vi "LV to ITX  Retrieve.vi"(0 "File or Folder Path":path=path "C:/", 5 "offset":i32, 7 "length":i32=1, 9 "index":T1={"A"=1, "B"=0, "C"=2, "D"=0, "E"=3, "N1"=0, "N2"=0, "N3"=0, "N4"=0}, 11 "stop":bool, 12 "file contains 2D data?":bool) -> (4 "A vs B":cluster{dbl[], dbl[]}[](graph)=[{[0.0624995231628418, 0.1406235694885254, 0.21874761581420898, 0.2968711853027344, 0.37499523162841797, 0.45311927795410156, 0.5468683242797852, 0.6249923706054688, 0.7031164169311523, 0.7812399864196777, 0.8593640327453613, 0.9374880790710449, 1.015612125396729, 1.109361171722412, 1.187485218048096, 1.265608787536621, 1.343732833862305, 1.437481880187988, 1.515605926513672, 1.578104972839355, 1.656229019165039, 1.749977588653564, 1.828101634979248, 1.906225681304932, 1.984349727630615, 2.062473773956299, 2.156222820281982, 2.234346389770508, 2.312470436096191, 2.390594482421875, 2.468718528747559, 2.546842575073242, 2.624966621398926, 2.703090667724609, 2.796839237213135, 2.874963283538818, 2.953087329864502, 3.031211376190186, 3.109335422515869, 3.187459468841553, 3.265583515167236, 3.359332084655762, 3.437456130981445, 3.515580177307129, 3.593704223632812, 3.671828269958496, 3.74995231628418, 3.843700885772705, 3.921824932098389, 3.999948978424072, 4.078073024749756, 4.156197071075439, 4.234321117401123, 4.312445163726807, 4.39056921005249, 4.484317779541016, 4.562441825866699, 4.640565872192383, 4.718689918518066, 4.79681396484375, 4.874938011169434, 4.968686580657959, 5.046810626983643, 5.124934673309326, 5.218683242797852, 5.296807289123535, 5.374931335449219, 5.453055381774902, 5.531179428100586, 5.60930347442627, 5.687427520751953, 5.781176090240479, 5.859300136566162, 5.937424182891846, 6.015548229217529, 6.093672275543213, 6.171796321868896, 6.24992036819458, 6.328044414520264, 6.421792984008789, 6.499917030334473, 6.578041076660156, 6.65616512298584, 6.734289169311523, 6.812413215637207, 6.906161785125732, 6.968660831451416, 7.0624098777771, 7.140533924102783, 7.218657970428467, 7.312406539916992, 7.390530586242676, 7.468654632568359, 7.546778678894043, 7.624902725219727, 7.70302677154541, 7.781150817871094, 7.859274387359619, 7.937398433685303, 8.015522480010986, 8.10927152633667, 8.187395572662354, 8.265519618988037, 8.343643188476562, 8.421767234802246, 8.49989128112793, 8.578015327453613, 8.671764373779297, 8.74988842010498, 8.828011989593506, 8.90613603591919, 8.984260082244873, 9.062384128570557, 9.14050817489624, 9.218632221221924, 9.31238079071045, 9.390504837036133, 9.468628883361816, 9.5467529296875, 9.624876976013184, 9.703001022338867, 9.78112506866455, 9.859249114990234, 9.95299768447876, 10.031121730804443], [0.0624995231628418, 0.1406235694885254, 0.21874761581420898, 0.2968711853027344, 0.37499523162841797, 0.45311927795410156, 0.5468683242797852, 0.6249923706054688, 0.7031164169311523, 0.7812399864196777, 0.8593640327453613, 0.9374880790710449, 1.015612125396729, 1.109361171722412, 1.187485218048096, 1.265608787536621, 1.343732833862305, 1.437481880187988, 1.515605926513672, 1.578104972839355, 1.656229019165039, 1.749977588653564, 1.828101634979248, 1.906225681304932, 1.984349727630615, 2.062473773956299, 2.156222820281982, 2.234346389770508, 2.312470436096191, 2.390594482421875, 2.468718528747559, 2.546842575073242, 2.624966621398926, 2.703090667724609, 2.796839237213135, 2.874963283538818, 2.953087329864502, 3.031211376190186, 3.109335422515869, 3.187459468841553, 3.265583515167236, 3.359332084655762, 3.437456130981445, 3.515580177307129, 3.593704223632812, 3.671828269958496, 3.74995231628418, 3.843700885772705, 3.921824932098389, 3.999948978424072, 4.078073024749756, 4.156197071075439, 4.234321117401123, 4.312445163726807, 4.39056921005249, 4.484317779541016, 4.562441825866699, 4.640565872192383, 4.718689918518066, 4.79681396484375, 4.874938011169434, 4.968686580657959, 5.046810626983643, 5.124934673309326, 5.218683242797852, 5.296807289123535, 5.374931335449219, 5.453055381774902, 5.531179428100586, 5.60930347442627, 5.687427520751953, 5.781176090240479, 5.859300136566162, 5.937424182891846, 6.015548229217529, 6.093672275543213, 6.171796321868896, 6.24992036819458, 6.328044414520264, 6.421792984008789, 6.499917030334473, 6.578041076660156, 6.65616512298584, 6.734289169311523, 6.812413215637207, 6.906161785125732, 6.968660831451416, 7.0624098777771, 7.140533924102783, 7.218657970428467, 7.312406539916992, 7.390530586242676, 7.468654632568359, 7.546778678894043, 7.624902725219727, 7.70302677154541, 7.781150817871094, 7.859274387359619, 7.937398433685303, 8.015522480010986, 8.10927152633667, 8.187395572662354, 8.265519618988037, 8.343643188476562, 8.421767234802246, 8.49989128112793, 8.578015327453613, 8.671764373779297, 8.74988842010498, 8.828011989593506, 8.90613603591919, 8.984260082244873, 9.062384128570557, 9.14050817489624, 9.218632221221924, 9.31238079071045, 9.390504837036133, 9.468628883361816, 9.5467529296875, 9.624876976013184, 9.703001022338867, 9.78112506866455, 9.859249114990234, 9.95299768447876, 10.031121730804443]}], 6 "C vs D":cluster{dbl[], dbl[]}[](graph)=[{[0.0624995231628418, 0.1406235694885254, 0.21874761581420898, 0.2968711853027344, 0.37499523162841797, 0.45311927795410156, 0.5468683242797852, 0.6249923706054688, 0.7031164169311523, 0.7812399864196777, 0.8593640327453613, 0.9374880790710449, 1.015612125396729, 1.109361171722412, 1.187485218048096, 1.265608787536621, 1.343732833862305, 1.437481880187988, 1.515605926513672, 1.578104972839355, 1.656229019165039, 1.749977588653564, 1.828101634979248, 1.906225681304932, 1.984349727630615, 2.062473773956299, 2.156222820281982, 2.234346389770508, 2.312470436096191, 2.390594482421875, 2.468718528747559, 2.546842575073242, 2.624966621398926, 2.703090667724609, 2.796839237213135, 2.874963283538818, 2.953087329864502, 3.031211376190186, 3.109335422515869, 3.187459468841553, 3.265583515167236, 3.359332084655762, 3.437456130981445, 3.515580177307129, 3.593704223632812, 3.671828269958496, 3.74995231628418, 3.843700885772705, 3.921824932098389, 3.999948978424072, 4.078073024749756, 4.156197071075439, 4.234321117401123, 4.312445163726807, 4.39056921005249, 4.484317779541016, 4.562441825866699, 4.640565872192383, 4.718689918518066, 4.79681396484375, 4.874938011169434, 4.968686580657959, 5.046810626983643, 5.124934673309326, 5.218683242797852, 5.296807289123535, 5.374931335449219, 5.453055381774902, 5.531179428100586, 5.60930347442627, 5.687427520751953, 5.781176090240479, 5.859300136566162, 5.937424182891846, 6.015548229217529, 6.093672275543213, 6.171796321868896, 6.24992036819458, 6.328044414520264, 6.421792984008789, 6.499917030334473, 6.578041076660156, 6.65616512298584, 6.734289169311523, 6.812413215637207, 6.906161785125732, 6.968660831451416, 7.0624098777771, 7.140533924102783, 7.218657970428467, 7.312406539916992, 7.390530586242676, 7.468654632568359, 7.546778678894043, 7.624902725219727, 7.70302677154541, 7.781150817871094, 7.859274387359619, 7.937398433685303, 8.015522480010986, 8.10927152633667, 8.187395572662354, 8.265519618988037, 8.343643188476562, 8.421767234802246, 8.49989128112793, 8.578015327453613, 8.671764373779297, 8.74988842010498, 8.828011989593506, 8.90613603591919, 8.984260082244873, 9.062384128570557, 9.14050817489624, 9.218632221221924, 9.31238079071045, 9.390504837036133, 9.468628883361816, 9.5467529296875, 9.624876976013184, 9.703001022338867, 9.78112506866455, 9.859249114990234, 9.95299768447876, 10.031121730804443], [1.78444e-07, 1.78444e-07, 1.78421e-07, 1.7837499999999998e-07, 1.7830699999999998e-07, 1.78239e-07, 1.7826199999999999e-07, 1.7835299999999998e-07, 1.7835299999999998e-07, 1.7837499999999998e-07, 1.7830699999999998e-07, 1.7826199999999999e-07, 1.7826199999999999e-07, 1.78284e-07, 1.78421e-07, 1.78444e-07, 1.78421e-07, 1.78421e-07, 1.7830699999999998e-07, 1.7830699999999998e-07, 1.7833e-07, 1.7835299999999998e-07, 1.7830699999999998e-07, 1.7830699999999998e-07, 1.78239e-07, 1.78171e-07, 1.78171e-07, 1.7826199999999999e-07, 1.7833e-07, 1.7833e-07, 1.7830699999999998e-07, 1.78193e-07, 1.78171e-07, 1.78171e-07, 1.78239e-07, 1.7826199999999999e-07, 1.78239e-07, 1.7821599999999999e-07, 1.78103e-07, 1.78125e-07, 1.78171e-07, 1.78239e-07, 1.78239e-07, 1.78193e-07, 1.7808000000000002e-07, 1.7808000000000002e-07, 1.78103e-07, 1.78193e-07, 1.78239e-07, 1.78239e-07, 1.78148e-07, 1.78103e-07, 1.78125e-07, 1.78239e-07, 1.78239e-07, 1.78239e-07, 1.78193e-07, 1.78103e-07, 1.78034e-07, 1.78057e-07, 1.78103e-07, 1.78148e-07, 1.78125e-07, 1.78103e-07, 1.78103e-07, 1.78034e-07, 1.77921e-07, 1.77943e-07, 1.78057e-07, 1.78103e-07, 1.7808000000000002e-07, 1.78057e-07, 1.77989e-07, 1.77921e-07, 1.78057e-07, 1.78034e-07, 1.78012e-07, 1.77989e-07, 1.77966e-07, 1.77852e-07, 1.77921e-07, 1.77966e-07, 1.77943e-07, 1.77943e-07, 1.77921e-07, 1.7783e-07, 1.77807e-07, 1.7783e-07, 1.77898e-07, 1.77989e-07, 1.77989e-07, 1.77989e-07, 1.77921e-07, 1.7783e-07, 1.77898e-07, 1.77921e-07, 1.77921e-07, 1.77898e-07, 1.77807e-07, 1.77761e-07, 1.77807e-07, 1.77921e-07, 1.77921e-07, 1.77943e-07, 1.77875e-07, 1.77807e-07, 1.77784e-07, 1.77875e-07, 1.77898e-07, 1.77921e-07, 1.77807e-07, 1.77761e-07, 1.77852e-07, 1.77875e-07, 1.77875e-07, 1.77875e-07, 1.77807e-07, 1.77739e-07, 1.77693e-07, 1.77784e-07, 1.77807e-07, 1.77784e-07, 1.77739e-07, 1.77693e-07, 1.77671e-07]}], 8 "E":dbl[][](graph)=[[172.002], [172.014], [172.02], [172.032], [172.05], [172.038], [171.99], [171.984], [172.008], [172.02], [172.038], [172.032], [172.008], [171.99], [171.984], [171.99], [172.008], [172.02], [172.032], [171.996], [172.002], [172.014], [172.032], [172.056], [172.056], [172.038], [172.008], [171.996], [172.014], [172.026], [172.032], [172.044], [172.008], [171.996], [171.99], [172.014], [172.032], [172.038], [172.032], [171.99], [171.984], [171.996], [172.014], [172.032], [172.026], [172.002], [171.99], [171.996], [172.02], [172.038], [172.05], [172.032], [172.002], [172.008], [172.014], [172.032], [172.044], [172.056], [172.044], [172.002], [171.996], [172.002], [172.026], [172.038], [172.044], [172.05], [172.02], [172.002], [171.99], [172.002], [172.008], [172.026], [172.02], [171.978], [171.978], [171.984], [171.99], [171.99], [172.002], [171.978], [171.96], [171.972], [171.984], [171.99], [171.996], [171.996], [171.978], [171.954], [171.948], [171.972], [171.99], [172.008], [172.032], [172.014], [171.996], [172.008], [172.014], [172.014], [172.008], [171.99], [171.972], [171.972], [171.99], [172.008], [172.032], [172.02], [171.996], [171.984], [171.996], [172.014], [172.02], [172.002], [171.972], [171.978], [171.99], [172.008], [172.026], [172.026], [171.99], [171.978], [171.99], [171.996], [172.002], [172.002], [172.002]], 10 "N":cluster{"N1":dbl, "N2":dbl, "N3":dbl, "N4":dbl}={"N1"=0.0624995231628418, "N2"=0.0624995231628418, "N3"=0.0624995231628418, "N4"=0.0624995231628418} {"N4" format="%#_6p"; "N3" format="%#_6p"; "N2" format="%#_6p"; "N1" format="%#_6p"}, 14 "Comments":string)   [LabVIEW 2016, in "LVtoITX.lvclass"]
uses:
  LVtoITX.lvclass
  <vilib>/Utility/miscctls.llb/LVOffsetAndMultiplierTypeDef.ctl
panel:
  in  "D  is time?":bool
  in  "B is time?":bool
  out "time":string[][](table)
  in  "Use Folder Index File?":bool
  in  "Generate Folder Index File?":bool
  in  "Ez name":string="Ez name"
  in  "Ey name":string="Ey name"
  in  "Ex name":string="Ex name"
  in  "C y name":string="C y name"
  in  "D x name":string="D x name"
  in  "A y name":string="A y name"
  in  "B x name":string="B x name"
  out "Index, Wavenames":string[][](table)
  in  "recolor traces?":bool
  in  "Ex":T2={"Offset"=0.0, "Multiplier"=1.0}
  in  "Ey":T2={"Offset"=0.0, "Multiplier"=1.0}
  out "Path":path
  out "counter":i32
  in  "pattern":string="*.itx"
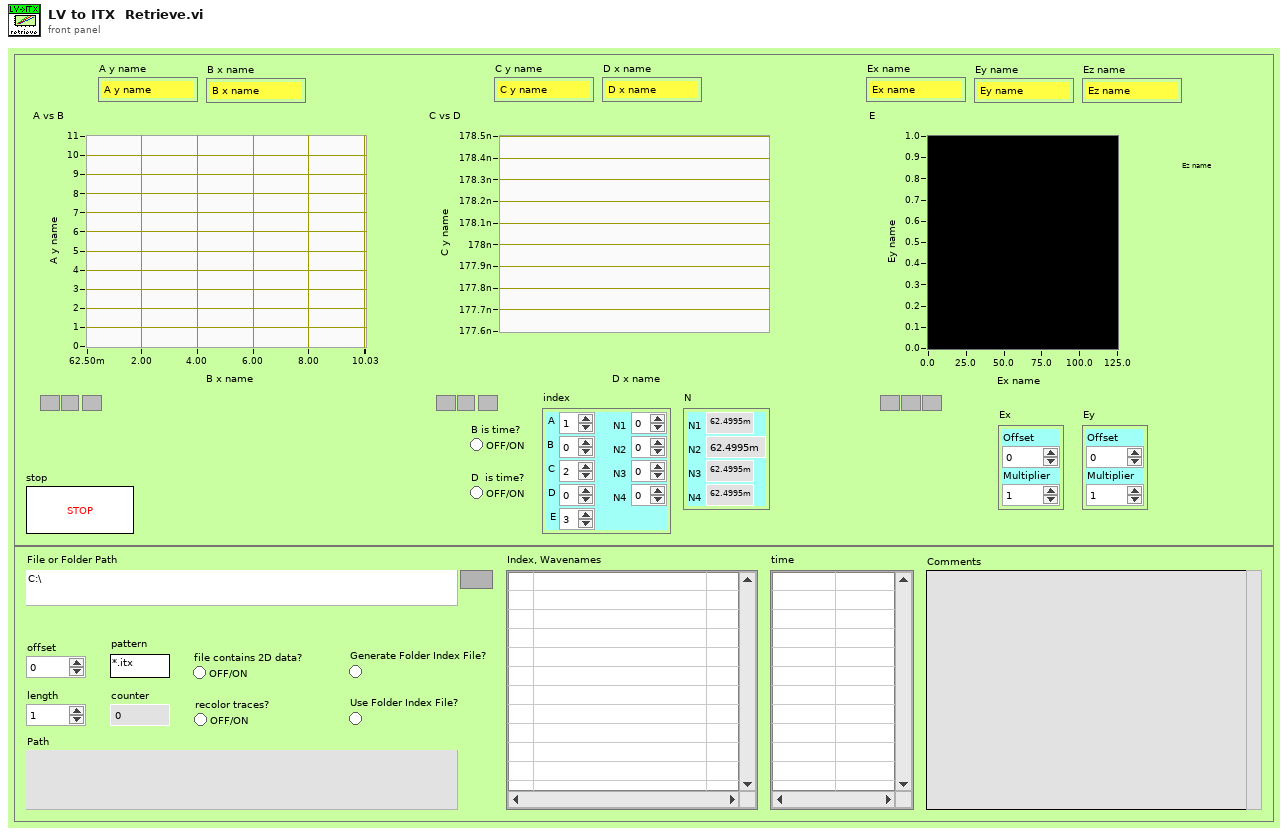
[diagram p1: front panel]
types:
  T1 = cluster{"A":i32, "B":i32, "C":i32, "D":i32, "E":i32, "N1":i32, "N2":i32, "N3":i32, "N4":i32}
  T2 = typedef "LVOffsetAndMultiplierTypeDef.ctl" = cluster{"Offset":dbl, "Multiplier":dbl}
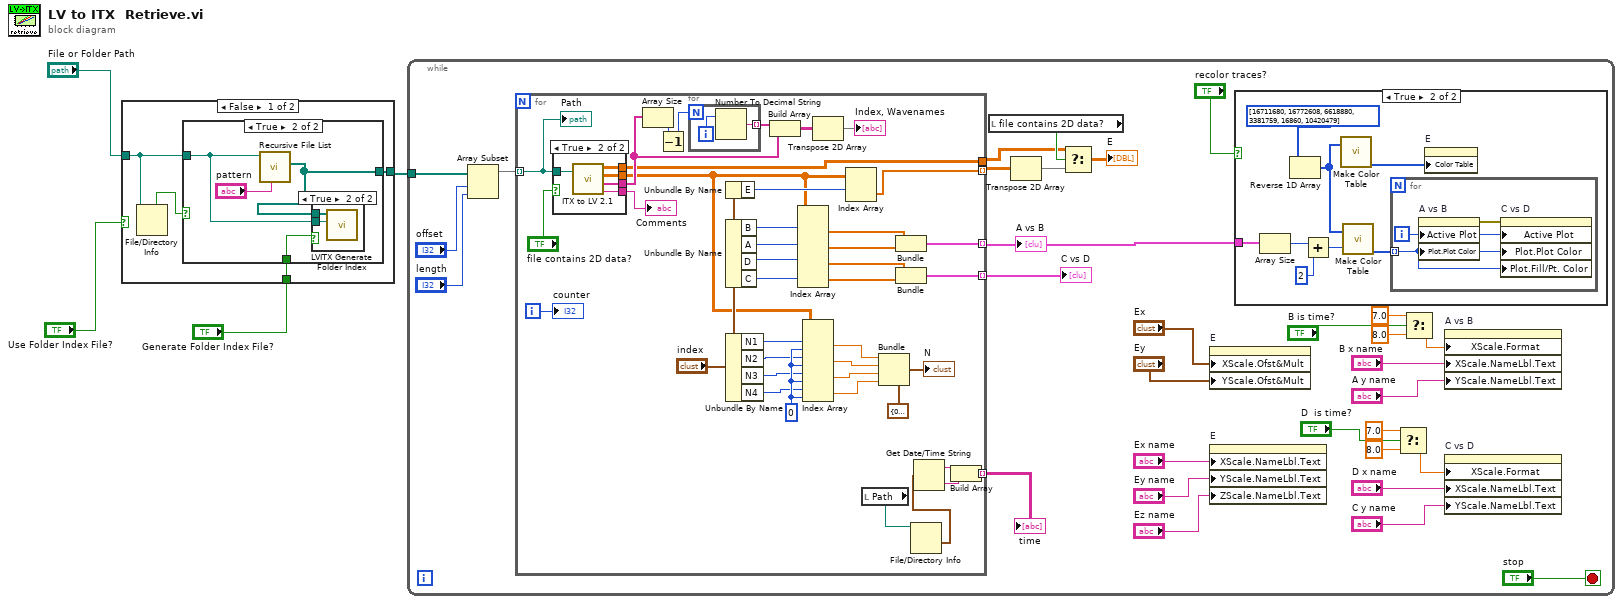
[diagram p0: block diagram]
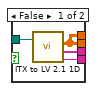
[diagram p3: hidden frame]
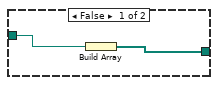
[diagram p4: hidden frame]
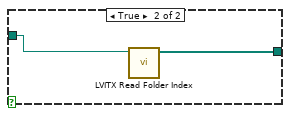
[diagram p6: hidden frame]
diagram:
  n1 = case shown="False" "Use Folder Index File?" {
    tunnel: [w6 w17] -> w2
    tunnel: "File or Folder Path" -> [w8 w18]
    tunnel: "Generate Folder Index File?" -> [w5 _]
    frame False {
      n2 = File/Directory Info(path=w8) -> (directory=w7:bool)  [unwired: 1 in, 6 out]
      n3 = case shown="True" w7 {
        tunnel: [w10 w13] -> w6
        tunnel: w8 -> [w9 w12]
        tunnel: w5 -> [_ w11]
        frame False {
          n4 = Build Array(w9) -> (w10:path[])
        }
        frame True {
          n5 = call <vilib>:"Recursive File List.vi"("pattern"="pattern", "Folder Path"=w12) -> ("All Files in Dir"=w13:path[])  [unwired: 5 in, 4 out]
          n6 = case shown="True" w11 {
            tunnel: w13 -> [_ w16]
            tunnel: w12 -> [_ w15]
            frame False {
            }
            frame True {
              n7 = call "LVITX Generate Folder Index.vi"("File or Folder Path"=w15, "All Files in Dir"=w16) -> ()  [unwired: 10 in]
            }
          }
        }
      }
    }
    frame True {
      n8 = call "LVITX Read Folder Index.vi"("File or Folder Path"=w18) -> ("Array"=w17:path[])  [unwired: 10 in]
    }
  }
  n9 = while {
    tunnel: w2 -> [w29]
    stop <- "stop" stop-if-true
    n10 = Array Subset(array=w29, index="offset", length="length") -> (w28:path[])
    n11 = for {
      tunnel: w28 -> [w99] mode=indexing
      tunnel: [w99] -> _ mode=indexing
      tunnel: [w98] -> w41 mode=indexing
      tunnel: [w96] -> w40 mode=indexing
      tunnel: [w73] -> w45 mode=indexing
      tunnel: [w87] -> w43
      tunnel: [w61] -> w32 mode=indexing
      i -> [w101]
      w86 = 0 ("disabled index (col)")
      n12 = case shown="True" "file contains 2D data?" {
        tunnel: [w107 w110] -> w100
        tunnel: [w105 w111] -> w65
        tunnel: w99 -> [w106 w112]
        tunnel: [w104 w109] -> w88
        tunnel: [w105 w108] -> w87
        frame False {
          n13 = call "ITX to LV 2.1 1D.vi"("file (use dialog)"=w106) -> ("1D arrays"=w105:dbl[][], "wave names"=w104:string[], "Notes"=w107:string)  [unwired: 2 in]
        }
        frame True {
          n14 = call "ITX to LV 2.1.vi"("file (use dialog)"=w112) -> ("2D array"=w108:dbl[][], "1D arrays"=w111:dbl[][], "wave names"=w109:string[], "Notes"=w110:string)  [unwired: 1 in]
        }
      }
      "Comments" <- w100
      n15 = Array Size(array=w88) -> (size(s)=w91:i32)
      n16 = Decrement(x=w91) -> (x-1=w90:i32)
      n17 = for {
        N: w90 -> [_]
        tunnel: [w102] -> w94 mode=indexing
        i -> [w103]
        n18 = Number To Decimal String(number=w103) -> (decimal integer string=w102:string)  [unwired: 1 in]
      }
      n19 = Unbundle By Name("index") -> ("E"=w78:i32)
      n20 = Unbundle By Name("index") -> ("B"=w77:i32, "A"=w76:i32, "D"=w75:i32, "C"=w74:i32)
      n21 = Unbundle By Name("index") -> ("N1"=w79:i32, "N2"=w80:i32, "N3"=w81:i32, "N4"=w82:i32)
      n22 = Build Array(w94, w88) -> (w89:string[][])
      n23 = Index Array(array=w65, index (row) #1=w77, index (row) #2=w76, index (row) #3=w75, index (row) #4=w74) -> (element #1=w70:dbl[], element #2=w69:dbl[], element #3=w92:dbl[], element #4=w95:dbl[])  [unwired: 4 in]
      n24 = Index Array(array=w65, index (row) #1=w79, index (col) #1=w86, index (row) #2=w80, index (col) #2=w86, index (row) #3=w81, index (col) #3=w86, index (row) #4=w82, index (col) #4=w86) -> (element #1=w66:dbl, element #2=w67:dbl, element #3=w68:dbl, element #4=w85:dbl)
      n25 = Transpose 2D Array(2D array=w89) -> (transposed array=→"Index, Wavenames":string[][])
      n26 = Index Array(array=w65, index (row)=w78) -> (element=w73:dbl[])  [unwired: 1 in]
      n27 = local read "Path"() -> (w71:path)
      n28 = Bundle(cluster=cluster{"N1":dbl, "N2":dbl, "N3":dbl, "N4":dbl} {"N1"=0.0, "N2"=0.0, "N3"=0.0, "N4"=0.0}, "N1"=w66, "N2"=w67, "N3"=w68, "N4"=w85) -> (→"N":cluster{"N1":dbl, "N2":dbl, "N3":dbl, "N4":dbl})
      n29 = Bundle("1D arrays"=w70, "1D arrays"=w69) -> (w98:cluster{"1D arrays":dbl[], "1D arrays":dbl[]})  [unwired: 1 in]
      n30 = Bundle("1D arrays"=w92, "1D arrays"=w95) -> (w96:cluster{"1D arrays":dbl[], "1D arrays":dbl[]})  [unwired: 1 in]
      n31 = File/Directory Info(path=w71) -> (last mod=w64:timestamp)  [unwired: 1 in, 6 out]
      n32 = Get Date/Time String(seconds (now)=w64) -> (date string=w63:string, time string=w62:string)  [unwired: 2 in]
      n33 = Build Array(w63, w62) -> (w61:string[])
      "counter" <- w101
      "Path" <- w99
    }
    "A vs B" <- w41
    "C vs D" <- w40
    "time" <- w32
    n34 = local read "file contains 2D data?"() -> (w48:bool)
    n35 = Transpose 2D Array(2D array=w45) -> (transposed array=w46:dbl[][])
    n36 = Select(t=w43, s=w48, f=w46) -> (s? t:f=→"E":dbl[][])
    n37 = property on="E" class="IntGraph (strict)"("XScale.Ofst&Mult"="Ex", "YScale.Ofst&Mult"="Ey") -> ()  [unwired: 2 in, 2 out]
    n38 = property on="E" class="IntGraph (strict)"("XScale.NameLbl.Text"="Ex name", "YScale.NameLbl.Text"="Ey name", "ZScale.NameLbl.Text"="Ez name") -> ()  [unwired: 2 in, 2 out]
    n39 = case shown="True" "recolor traces?" {
      tunnel: w41 -> [_ w52]
      frame False {
      }
      frame True {
        n40 = Array Size(array=w52) -> (size(s)=w53:i32)
        n41 = Reverse 1D Array(array=u32[] [16711680, 16772608, 6618880, 3381759, 16860, 10420479] ("color scale")) -> (reversed array=w51:u32[])
        n42 = Add(x=w53, y=2 ("x")) -> (x+y=w57:i32)
        n43 = call <userlib>:"Make Color Table.vi"("Array"=w51) -> ("Color Tbl"=w55:u32[])  [unwired: 1 in, 3 out]
        n44 = call <userlib>:"Make Color Table.vi"("Array"=w51, "Size/3"=w57) -> ("Color Tbl"=w54:u32[])  [unwired: 3 out]
        n45 = for {
          tunnel: w54 -> [w58] mode=indexing
          i -> [w59]
          n46 = property on="A vs B" class="XYGraph (strict)"("Active Plot"=w59, "Plot.Plot Color"=w58) -> (error out=w60:errorcluster)  [unwired: 2 in, 1 out]
          n47 = property on="C vs D" class="XYGraph (strict)"(error in=w60, "Active Plot"=w59, "Plot.Plot Color"=w58, "Plot.Fill/Pt. Color"=w58) -> ()  [unwired: 1 in, 2 out]
        }
        n48 = property on="E" class="IntGraph (strict)"("Color Table"=w55) -> ()  [unwired: 2 in, 2 out]
      }
    }
    n49 = Select(t=7.0, s="D  is time?", f=8.0) -> (s? t:f=w24:dbl)
    n50 = Select(t=7.0, s="B is time?", f=8.0) -> (s? t:f=w25:dbl)
    n51 = property on="A vs B" class="XYGraph (strict)"("XScale.Format"=w25, "XScale.NameLbl.Text"="B x name", "YScale.NameLbl.Text"="A y name") -> ()  [unwired: 2 in, 2 out]
    n52 = property on="C vs D" class="XYGraph (strict)"("XScale.Format"=w24, "XScale.NameLbl.Text"="D x name", "YScale.NameLbl.Text"="C y name") -> ()  [unwired: 2 in, 2 out]
  }
